vi "Circular Buffer (array).vi"(6 "History Length [1024]":i32=1024, 7 "reset":bool, 8 "error in":errorcluster, 11 "Array in":dbl[](array[numeric])) -> (0 "error out":errorcluster, 3 "Array out":dbl[](array[numeric]))   [LabVIEW 2019, in "xy_utilities.lvlib"]
doc: "Circular Buffer with controllable reset and history length."
uses:
  xy_utilities.lvlib
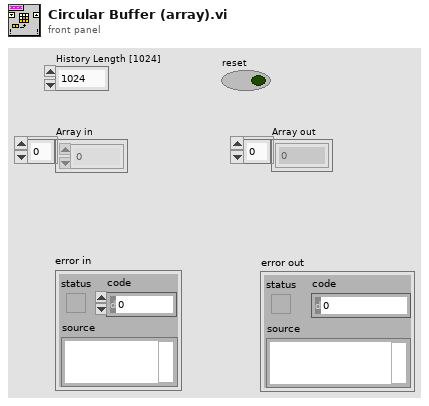
[diagram p1: front panel]
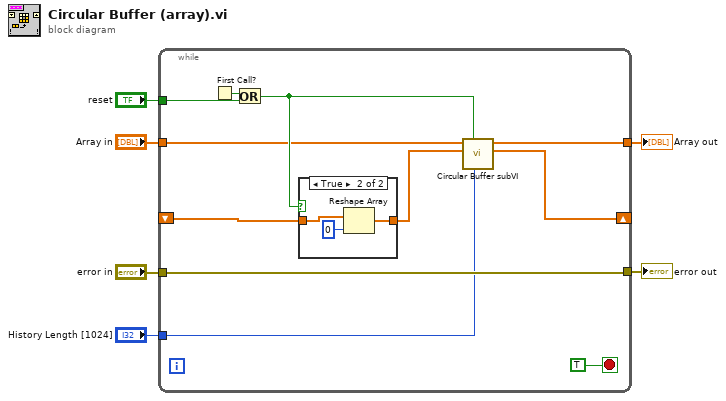
[diagram p0: block diagram]
diagram:
  n1 = while {
    tunnel: "Array in" -> [w7]
    tunnel: [w17] -> w5
    tunnel: "error in" -> [w17]
    tunnel: "reset" -> [w15]
    shift-right: [w11] -> _
    shift-left: _ -> [w9]
    tunnel: [w12] -> w2
    tunnel: "History Length [1024]" -> [w13]
    stop <- TRUE stop-if-true
    n2 = First Call?() -> (First Call?: T/F=w16:bool)
    n3 = Or(x=w16, y=w15) -> (x .or. y?=w10:bool)
    n4 = case shown="True" w10 {
      tunnel: w9 -> [w18 w19]
      tunnel: [w18 w20] -> w8
      frame False {
      }
      frame True {
        n5 = Reshape Array(w19, 0 ("dimension size")) -> (w20:dbl[])
      }
    }
    n6 = call "Circular Buffer subVI.vi"("History Length [1024]"=w13, "Reset"=w10, "Buffer in"=w8, "Array in"=w7) -> ("Buffer out"=w11:dbl[], "Array out"=w12:dbl[])  [unwired: 6 in]
  }
  "Array out" <- w2
  "error out" <- w5
